vi "Sandbox2.vi"   [LabVIEW 2014]
uses:
  Topic Child Classes/Launch Client/Launch Client.lvclass
  Architecture/Classes/Client_class/Client.lvclass
  Client Child Classes/Client Manager/Client Manager.lvclass
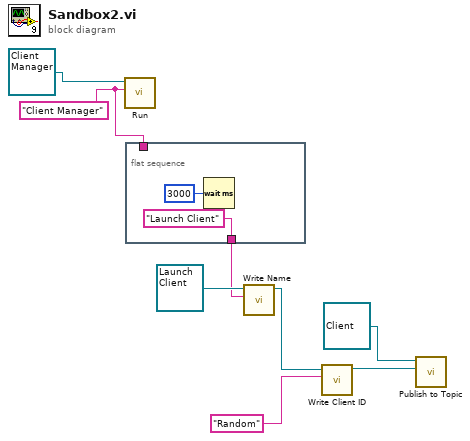
[diagram p0: block diagram]
diagram:
  w2 = "Client Manager" ("ID")
  n1 = call-dynamic "Run.vi"("ID"=w2, "Client in"=refnum<class "Client Manager.lvclass"> refnum ("Client Manager.lvclass")) -> ()  [unwired: 8 in, 2 out]
  n2 = flat-sequence {
    tunnel: w2 -> [_]
    tunnel: ["Launch Client" ("Name")] -> w1
    frame #0 {
      n3 = Wait (ms)(milliseconds to wait=u32 3000) -> ()  [unwired: 1 out]
    }
  }
  n4 = call-dynamic "Write Name.vi"("Name"=w1, "Topic in"=refnum<class "Launch Client.lvclass"> refnum ("Launch Client.lvclass")) -> ("Topic out"=w5:refnum<class "Launch Client.lvclass">)  [unwired: 8 in, 1 out]
  n5 = call-dynamic "Write Client ID.vi"("Client ID"="Random", "Launch Client in"=w5) -> ("Launch Client out"=w6:refnum<class "Launch Client.lvclass">)  [unwired: 8 in, 1 out]
  n6 = call-dynamic "Publish to Topic.vi"("Topic.lvclass"=w6, "Client in"=refnum<class "Client.lvclass"> refnum ("Client.lvclass")) -> ()  [unwired: 8 in, 2 out]
